vi "LatestDataTimeStamp.vi"(7 "Action":enum16{"Set", "Get"}(ring), 8 "error in (no error)":errorcluster, 10 "TimeStamp":timestamp, 11 "Plugin Name":string) -> (0 "error IO":errorcluster, 2 "Latest Data Timestamp":timestamp, 3 "Plugin Name out":string)   [LabVIEW 2018, in "AcPwrPlugins.lvlib" / "AcPwrBase.lvclass"]
uses:
  AcPwrBase.lvclass
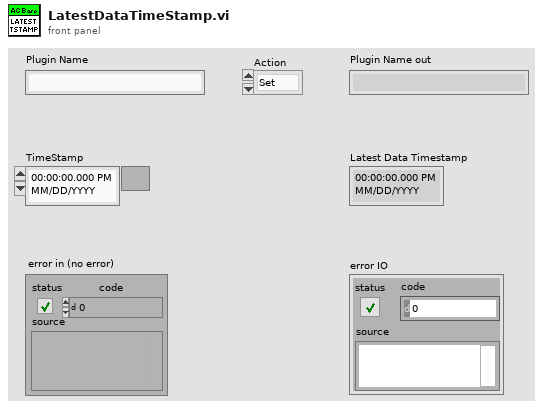
[diagram p1: front panel]
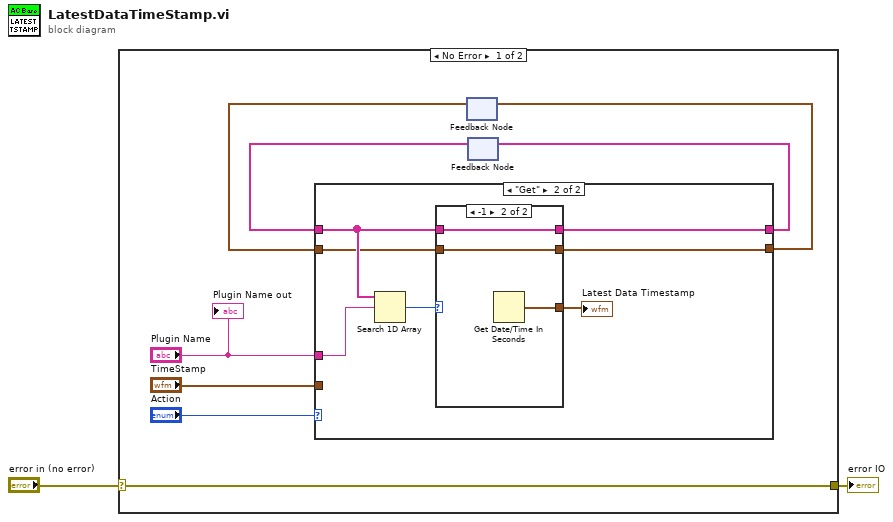
[diagram p0: block diagram]
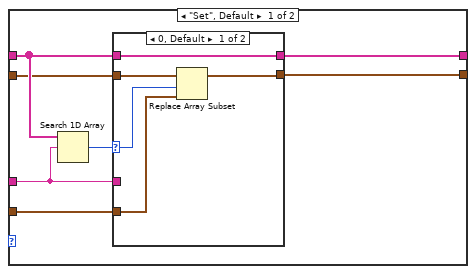
[diagram p2: hidden frame]
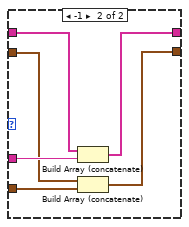
[diagram p3: hidden frame]
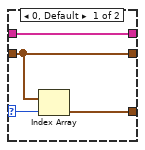
[diagram p4: hidden frame]
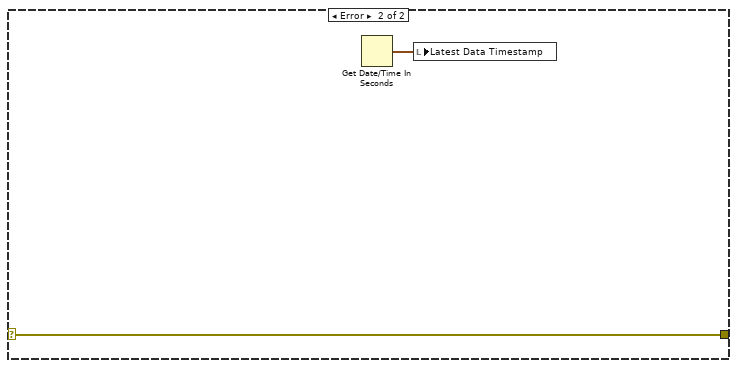
[diagram p5: hidden frame]
diagram:
  n1 = case shown="No Error" "error in (no error)" {
    selector: "error in (no error)" -> [w3 w44]
    tunnel: [w3 w44] -> w1
    frame No Error {
      n2 = feedback #1() -> (w4:timestamp[])  [unwired: 1 in]
      n3 = feedback #2() -> (w6:string[])  [unwired: 1 in]
      n4 = case shown="\"Get\"" "Action" {
        tunnel: "Plugin Name" -> [w14 w35]
        tunnel: "TimeStamp" -> [w13 _]
        tunnel: [w17 w33] -> w7
        tunnel: w6 -> [w16 w34]
        tunnel: [w12 w31] -> w5
        tunnel: w4 -> [w11 w32]
        frame "Set", Default {
          n5 = Search 1D Array(1D array=w16, element=w14) -> (index of element=w15:i32)  [unwired: 1 in]
          n6 = case shown="0, Default" w15 {
            selector: w15 -> [w19 _]
            tunnel: w14 -> [_ w28]
            tunnel: [w22 w26] -> w17
            tunnel: w16 -> [w22 w27]
            tunnel: w13 -> [w20 w25]
            tunnel: [w18 w24] -> w12
            tunnel: w11 -> [w21 w23]
            frame 0, Default {
              n7 = Replace Array Subset(array=w21, new element=w20, index=w19) -> (w18:timestamp[])
            }
            frame -1 {
              n8 = Build Array (concatenate)(w27, w28) -> (w26:string[])
              n9 = Build Array (concatenate)(w23, w25) -> (w24:timestamp[])
            }
          }
        }
        frame "Get" {
          n10 = Search 1D Array(1D array=w34, element=w35) -> (index of element=w30:i32)  [unwired: 1 in]
          n11 = case shown="-1" w30 {
            selector: w30 -> [w37 _]
            tunnel: w34 -> [w39 w42]
            tunnel: [w39 w42] -> w33
            tunnel: w32 -> [w38 w41]
            tunnel: [w38 w41] -> w31
            tunnel: [w36 w40] -> w29
            frame 0, Default {
              n12 = Index Array(array=w38, index=w37) -> (element=w36:timestamp)
            }
            frame -1 {
              n13 = Get Date/Time In Seconds() -> (seconds since 1Jan1904=w40:timestamp)
            }
          }
          "Latest Data Timestamp" <- w29
        }
      }
      n14 = feedback-in #1(w5) -> ()
      n15 = feedback-in #2(w7) -> ()
      "Plugin Name out" <- "Plugin Name"
    }
    frame Error {
      n16 = Get Date/Time In Seconds() -> (seconds since 1Jan1904=w43:timestamp)
      n17 = local write "Latest Data Timestamp"(w43) -> ()
    }
  }
  "error IO" <- w1
